vi "Calculator-teardown.vi"(8 "error out":errorcluster, 10 "result":dbl, 11 "test case ID":string) -> (3 "result":bool)   [LabVIEW 2018]
doc: "The teardown VI should be executed after the VI under test in the harness VI. In this VI you can evaluate the outputs of the VI under test.\n\nSee the Help Document for more information. (<b>Help</b> > <b>IncQuery Labs</b> > <b>InstaCoverage</b> > <b>InstaCoverage Help...</b>)"
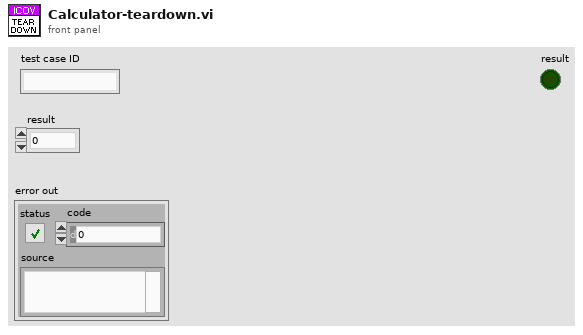
[diagram p1: front panel]
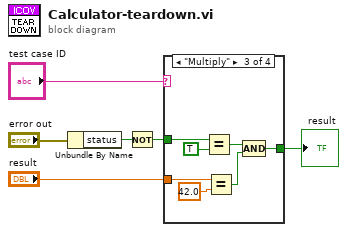
[diagram p0: block diagram]
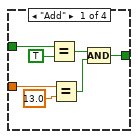
[diagram p2: hidden frame]
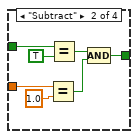
[diagram p3: hidden frame]
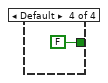
[diagram p4: hidden frame]
diagram:
  n1 = Unbundle By Name("error out") -> ("status"=w3:bool)
  n2 = Not(x=w3) -> (.not. x?=w1:bool)
  n3 = case shown="\"Multiply\"" "test case ID" {
    tunnel: [w7 w14 w21 FALSE] -> w5
    tunnel: "result" -> [w13 w20 w27 _]
    tunnel: w1 -> [w11 w18 w25 _]
    frame "Add" {
      n4 = Equal?(x=w11, y=TRUE) -> (x = y?=w9:bool)
      n5 = Equal?(x=w13, y=13.0) -> (x = y?=w8:bool)
      n6 = Compound Arithmetic op=AND(w9, w8) -> (w7:bool)
    }
    frame "Subtract" {
      n7 = Equal?(x=w20, y=1.0) -> (x = y?=w15:bool)
      n8 = Equal?(x=w18, y=TRUE) -> (x = y?=w16:bool)
      n9 = Compound Arithmetic op=AND(w16, w15) -> (w14:bool)
    }
    frame "Multiply" {
      n10 = Equal?(x=w25, y=TRUE) -> (x = y?=w23:bool)
      n11 = Equal?(x=w27, y=42.0) -> (x = y?=w22:bool)
      n12 = Compound Arithmetic op=AND(w23, w22) -> (w21:bool)
    }
    frame Default {
    }
  }
  "result" <- w5
